vi "配置初始化.vi"(8 "error in (no error)":errorcluster) -> (0 "error out":errorcluster)   [LabVIEW 2022 SP3, in "斯坦道总氮V2.lvlib"]
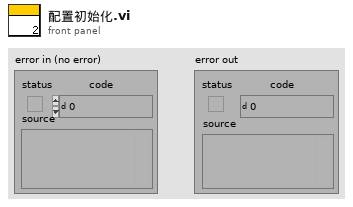
[diagram p1: front panel]
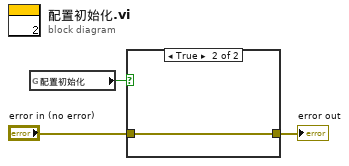
[diagram p0: block diagram]
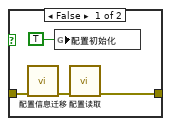
[diagram p2: hidden frame]
diagram:
  n1 = global read "VAR总磷总氮全局变量.vi" "配置初始化"() -> (w1:bool)
  n2 = case shown="True" w1 {
    tunnel: "error in (no error)" -> [w6 w8]
    tunnel: [w5 w8] -> w2
    frame False {
      n3 = call "配置信息迁移.vi"("error in (no error)"=w6) -> ("error out"=w7:errorcluster)  [unwired: 10 in]
      n4 = global write "VAR总磷总氮全局变量.vi" "配置初始化"(TRUE ("配置初始化")) -> ()
      n5 = call "配置读取.vi"("error in (no error)"=w7) -> ("error out"=w5:errorcluster)  [unwired: 10 in]
    }
    frame True {
    }
  }
  "error out" <- w2
